vi "ImaqToPicture.vi"(8 "error in (no error)":errorcluster, 10 "Image":T1) -> (0 "error out":errorcluster, 2 "Picture":picture)   [LabVIEW 2017]
uses:
  <vilib>/vision/Image Controls.llb/IMAQ Image.ctl
  <vilib>/picture/picture.llb/Draw True-Color Pixmap.vi
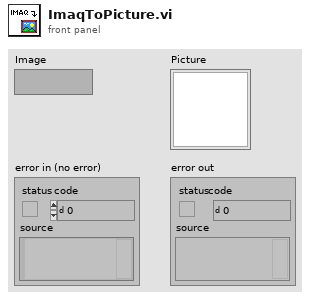
[diagram p1: front panel]
types:
  T1 = typedef "IMAQ Image.ctl" = refnum<image>
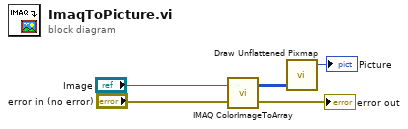
[diagram p0: block diagram]
diagram:
  n1 = call "IMAQ ColorImageToArray"("Image"="Image", "error in (no error)"="error in (no error)") -> ("Image Pixels (U32)"=w4:u32[][], "error out"=→"error out":errorcluster)  [unwired: 2 in, 1 out]
  n2 = call-poly <vilib>:"Draw Unflattened Pixmap.vi"("data (RGB format)"=w4) -> ("new picture"=→"Picture":picture)  [unwired: 8 in]
